vi "qONL.vi"(0 "System no.":i32=1 min=1 max=4 step=1, 2 "Channels to query":string[](array[string]), 3 "All channels?":bool=TRUE, 5 "error in":errorcluster) -> (14 "Online status?":bool, 15 "Online status (Array)?":bool[](array[boolean]), 19 "error out":errorcluster)   [LabVIEW 2020]
doc: "Indicates whether system is online (TRUE) or offline (FALSE). GCS 1.0: Online status is valid for all channels/axes of the system. GCS 2.0: Online status is channel specific.\n\nE-516: All channels? must be TRUE. Online status (Array)? is not valid, Online status? contains online status for all channels/axes.\nE-517, E-518: All channels? must be FALSE. Online status is channel specific."
panel:
  # "Indicates whether system is online (TRUE) or offline (FALSE). GCS1.0: Online status is valid for all\nchannels/axes of the system. GCS2.0: Online status is channel specific."
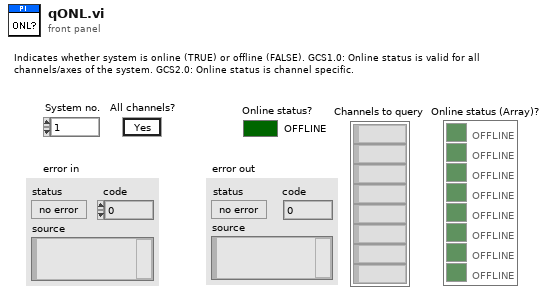
[diagram p1: front panel]
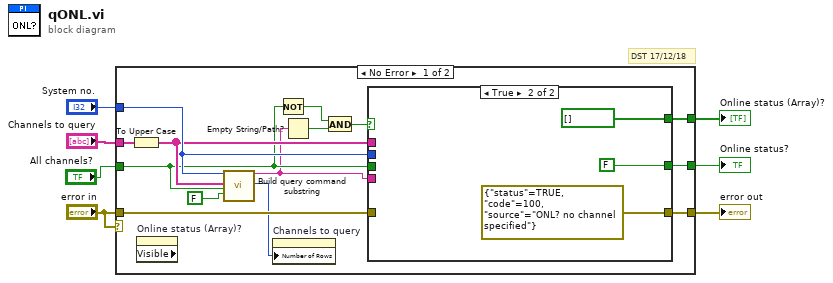
[diagram p0: block diagram]
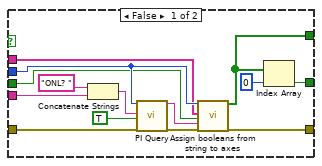
[diagram p2: hidden frame]
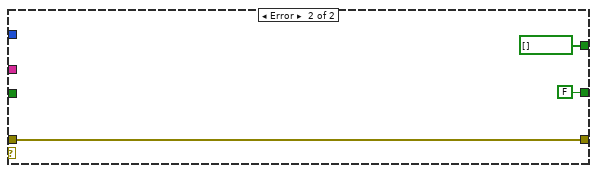
[diagram p3: hidden frame]
diagram:
  # "DST 17/12/18"
  n1 = case shown="No Error" "error in" {
    tunnel: "error in" -> [w21 w41]
    tunnel: [w20 FALSE ("Boolean")] -> w7
    tunnel: "Channels to query" -> [w18 _]
    tunnel: "System no." -> [w16 _]
    tunnel: [w14 w41] -> w4
    tunnel: [w13 bool[] [] ("Booleans")] -> w3
    tunnel: "All channels?" -> [w11 _]
    frame No Error {
      n2 = To Upper Case(1:w18) -> (0:w12:string[])
      n3 = property on="Online status (Array)?" class="Arr (strict)" props=["Visible"]() -> ()  [unwired: 2 in, 3 out]
      n4 = call "Build query command substring.vi"("System no."=w16, "Axes to query in"=w12, "Query\nAll axes?"=w11, "For all axes: use\nAxis identifier?"=FALSE ("For all axes: use\nAxis identifier?")) -> ("Command substring"=w9:string, "Number of rows"=w10:u32)  [unwired: 2 in, 12 out]
      n5 = property on="Channels to query" class="Arr (strict)"("Number of Rows"=w10) -> ()  [unwired: 2 in, 2 out]
      n6 = Not(x=w11) -> (.not. x?=w19:bool)
      n7 = Empty String/Path?(string/path=w9) -> (empty?=w8:bool)
      n8 = And(x=w19, y=w8) -> (x .and. y?=w15:bool)
      n9 = case shown="True" w15 {
        tunnel: w21 -> [w35 _]
        tunnel: [w24 FALSE] -> w20
        tunnel: w9 -> [w32 _]
        tunnel: w16 -> [w30 _]
        tunnel: [w27 errorcluster {"status"=TRUE, "code"=100, "source"="ONL? no channel specified"} ("error out")] -> w14
        tunnel: [w26 bool[] [] ("Booleans")] -> w13
        tunnel: w12 -> [w29 _]
        tunnel: w11 -> [w28 _]
        frame False {
          n10 = Concatenate Strings("ONL? ", w32) -> (w31:string)
          n11 = call "PI Query.vi"("System no."=w30, "String to send"=w31, "Attach termination char.?"=TRUE ("Attach Linefeed?"), "error in"=w35) -> ("String read"=w23:string, "error out"=w22:errorcluster)  [unwired: 3 in, 11 out]
          n12 = call "Assign booleans from string to axes.vi"("System no."=w30, "Queried axes"=w29, "All axes queried?"=w28, "Input String"=w23, "error in"=w22) -> ("Booleans"=w26:bool[], "error out"=w27:errorcluster)  [unwired: 13 out]
          n13 = Index Array(array=w26, index=0) -> (element=w24:bool)
        }
        frame True {
        }
      }
    }
    frame Error {
    }
  }
  "Online status?" <- w7
  "Online status (Array)?" <- w3
  "error out" <- w4
